vi "read.vi"() -> ()   [LabVIEW 2013]
panel:
  out "Affichage des erreurs":string
  out "Affichage du code":string
  out "Pixmap depuis la source":string
  in  "color 1":i32
  in  "Nombre de couleur":i32
  in  "Fichier .m":path
  in  "Valider":bool
  in  "Valider":bool
  in  "Fichier txt":path
  out "Pixmap.txt":string
  out "courbes.m":string
  in  "Pixmap":i32[][](array[numeric])
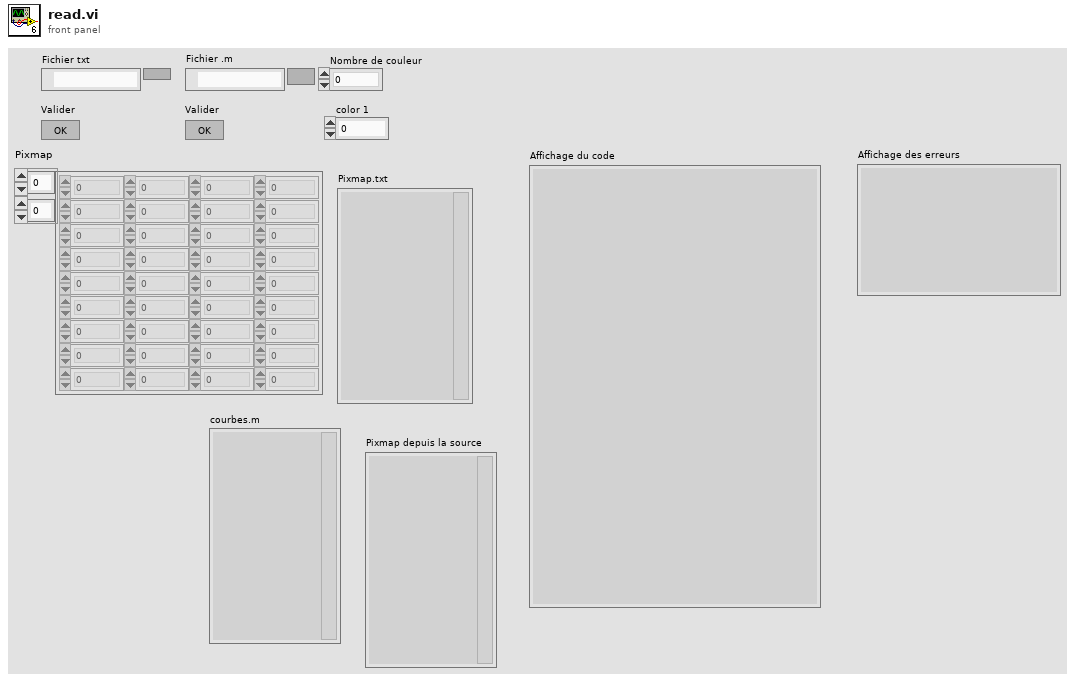
[diagram p1: front panel]
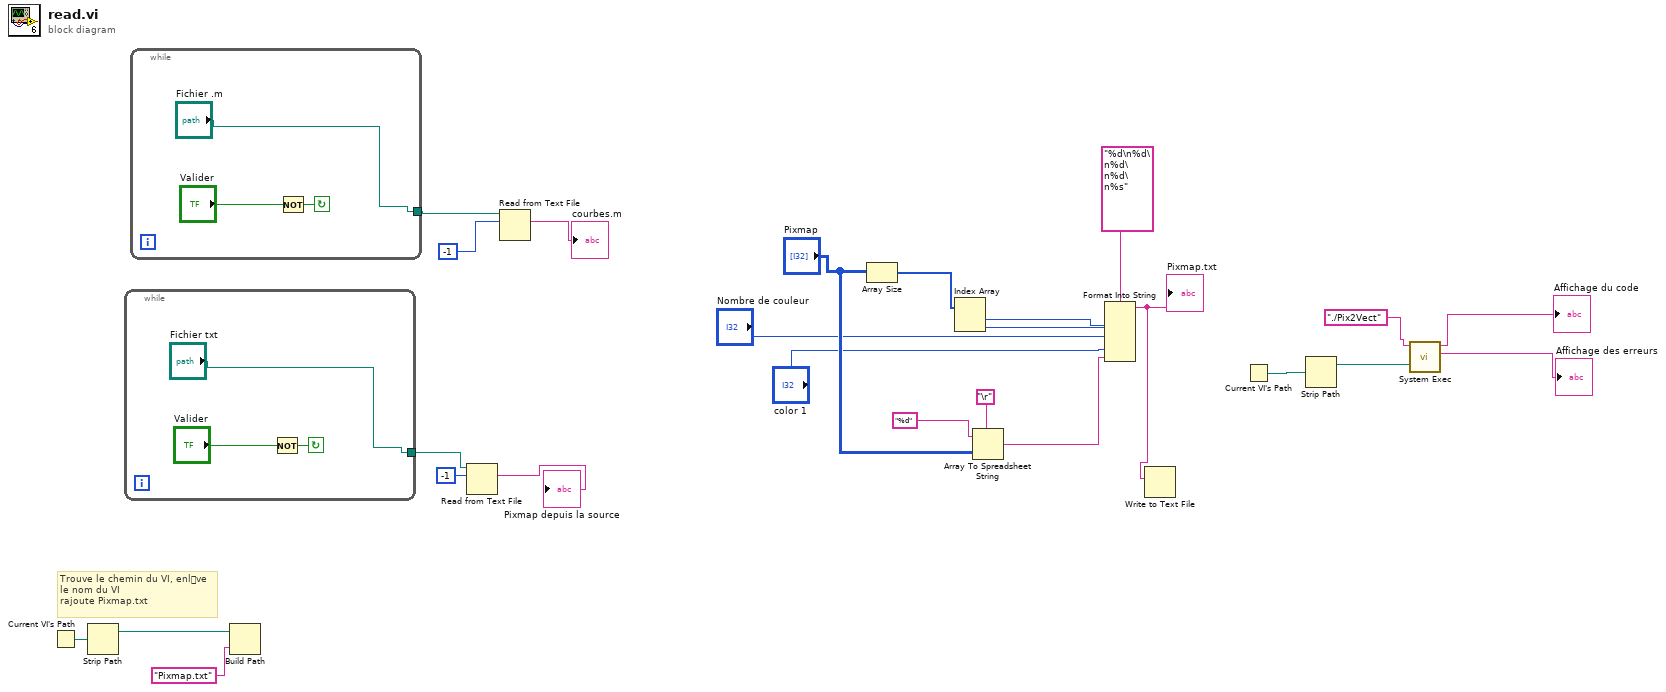
[diagram p0: block diagram]
diagram:
  # "Trouve le chemin du VI, enlve le nom du VI \nrajoute Pixmap.txt"
  n1 = Current VI's Path() -> (path=w24:path)
  n2 = Strip Path(path=w24) -> (stripped path=w22:path)  [unwired: 1 out]
  n3 = while {
    tunnel: ["Fichier txt"] -> w21
    stop <- w26 continue-if-true
    n4 = Not(x="Valider") -> (.not. x?=w26:bool)
  }
  n5 = while {
    tunnel: ["Fichier .m"] -> w18
    stop <- w29 continue-if-true
    n6 = Not(x="Valider") -> (.not. x?=w29:bool)
  }
  n7 = Build Path(base path=w22, name or relative path="Pixmap.txt") -> ()  [unwired: 1 out]
  n8 = Read from Text File(file (use dialog)=w21, count=-1) -> (text=→"Pixmap depuis la source":string)  [unwired: 2 in, 3 out]
  n9 = Read from Text File(file (use dialog)=w18, count=-1) -> (text=→"courbes.m":string)  [unwired: 2 in, 3 out]
  n10 = Array Size(array="Pixmap") -> (size(s)=w14:i32[])
  n11 = Index Array(array=w14) -> (element #1=w13:i32, element #2=w12:i32)  [unwired: 2 in]
  n12 = Array To Spreadsheet String(delimiter (Tab)="\r", array="Pixmap", 3:"%d") -> (spreadsheet string=w7:string)
  n13 = Format Into String(format string="%d\n%d\n%d\n%d\n%s", w13, w12, "Nombre de couleur", "color 1", w7) -> (resulting string=w1:string)  [unwired: 2 in, 1 out]
  "Pixmap.txt" <- w1
  n14 = Write to Text File(text=w1) -> ()  [unwired: 3 in, 3 out]
  n15 = Current VI's Path() -> (path=w5:path)
  n16 = Strip Path(path=w5) -> (stripped path=w6:path)  [unwired: 1 out]
  n17 = call <vilib>:"System Exec.vi"("working directory"=w6, "command line"="./Pix2Vect") -> ("standard error"=→"Affichage des erreurs":string, "standard output"=→"Affichage du code":string)  [unwired: 6 in, 2 out]
